vi "DynamicHoppingScan.vi"() -> ()   [LabVIEW 2014]
uses:
  <vilib>/userdefined/High Color/nirio_resource_hc.ctl
  <vilib>/Instr/_visa.llb/VISA Configure Serial Port (Instr).vi
  <vilib>/FPGAPlugInAG/PCIe-7851R/niLvFpga_Open_PCIe-7851R.vi
  <vilib>/rvi/interface/common/dynamic/niFpgaDynamicAddResources.vi
  <vilib>/Utility/error.llb/Error Cluster From Error Code.vi
  <vilib>/rvi/errors/niLvFpgaAdjustHostInterfaceError.vi
  <vilib>/FPGAPlugInAG/Dynamic/niLvFpga_Close_Dynamic.vi
  <vilib>/rvi/interface/nirviOpenFPGA/nirviOpenFPGA.xnode
  FPGATest_FPGATarget_PIZApproaching_ngy2QjQf4ns.lvbitx
  <vilib>/rvi/interface/nirviReadWriteControl/nirviReadWriteControl.xnode
  <vilib>/rvi/interface/nirviCloseFPGA/nirviCloseFPGA.xnode
  FPGATest_FPGATarget_PIZWithdraw_LXoQbY-wYvI.lvbitx
  <vilib>/rvi/interface/Simulation/niFpgaSimulationCallBeginRW.vi
  NiFpgaLv.dll
  NextXYPos.dll
panel:
  out "RoughXYZErr?":string
  out "XY Graph":cluster{dbl[], dbl[]}(graph)
  in  "stepMultiplier / 0.305nm":i16
  out "preCurrIndexDia":i16(graph)
  out "PIZPosDia":i16(graph)
  out "PIZPos":i16
  out "preCurrIndex":i16
  out "refCurrIndex":i16
  in  "stop":bool
  in  "ThresholdIndex":i32
  in  "PIZ":T1
  in  "PIZRisingLimitLen / um":dbl
  out "YPos?":dbl
  out "XPos?":dbl
  in  "YIStep / um":dbl format="%#_13g"
  in  "XIStep / um":dbl format="%#_13g"
  in  "YDirTotalLength / um":dbl format="%#_13g"
  in  "XDirTotalLength / um":dbl format="%#_13g"
  in  "Y Init / um":dbl format="%#_13g"
  in  "X Init / um":dbl format="%#_13g"
  in  "AllLoopSleep ms":i32
  in  "RoughXYZ":refnum<visa-resource-name>
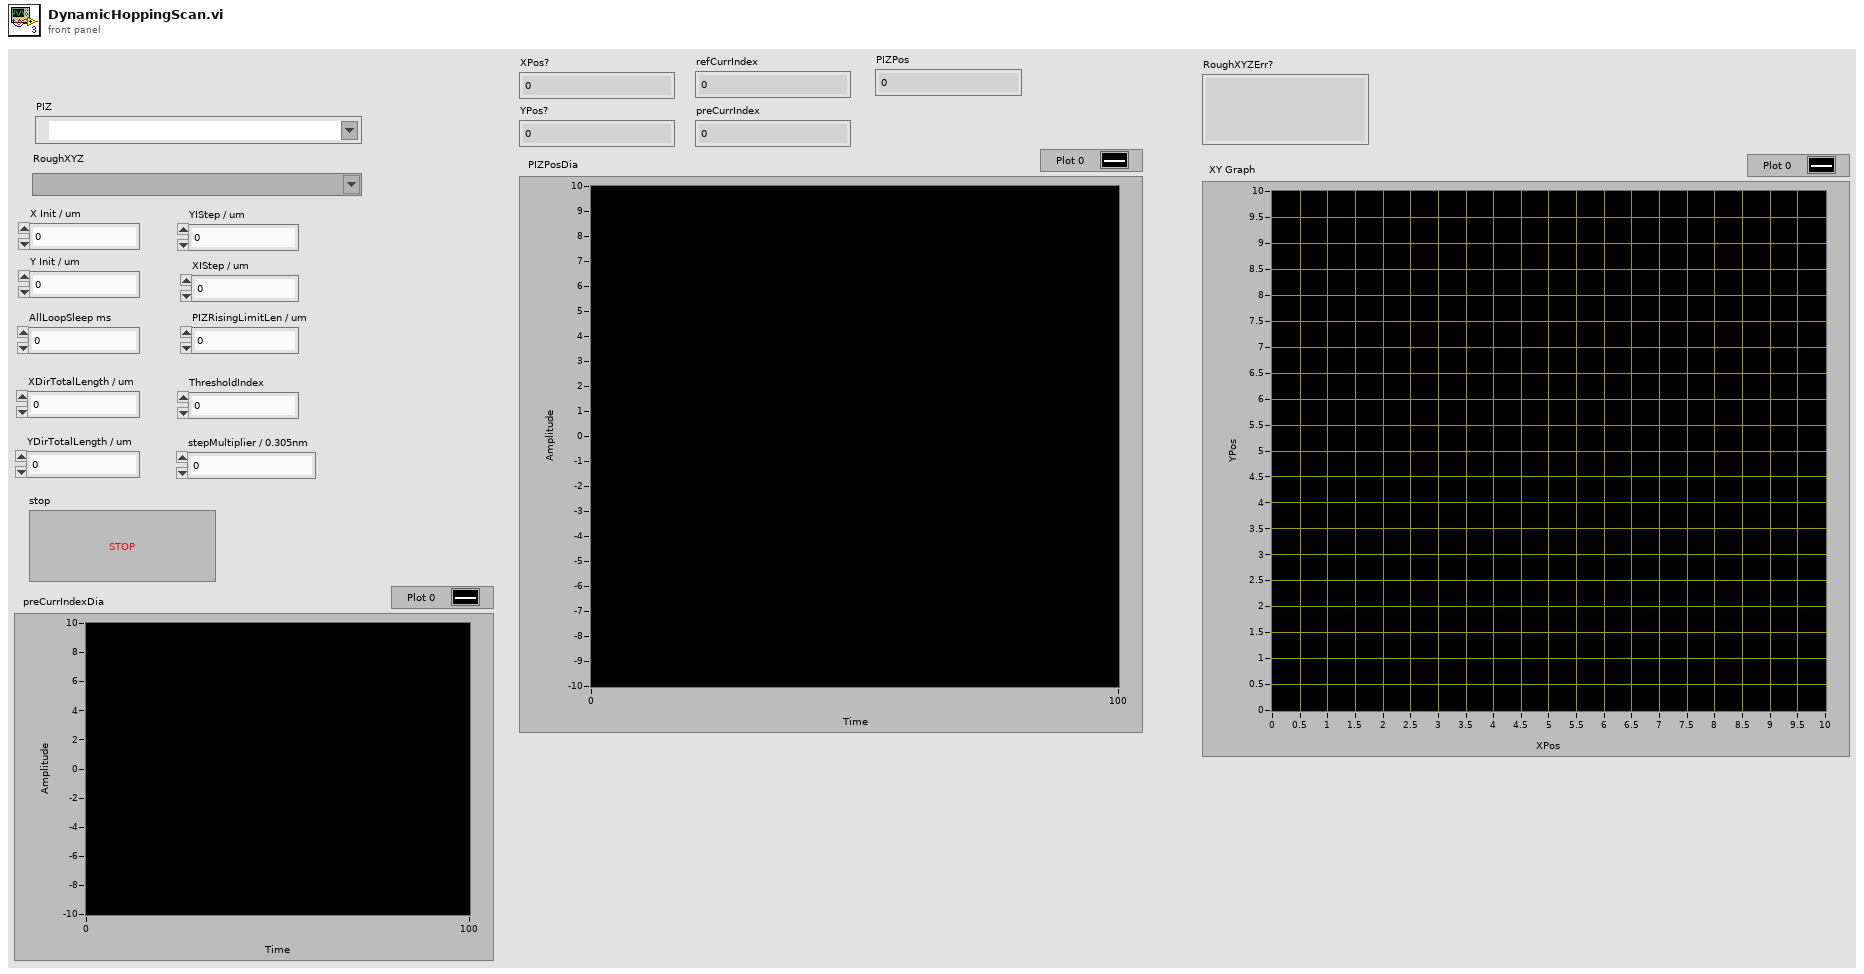
[diagram p1: front panel]
types:
  T1 = typedef "nirio_resource_hc.ctl" = tag
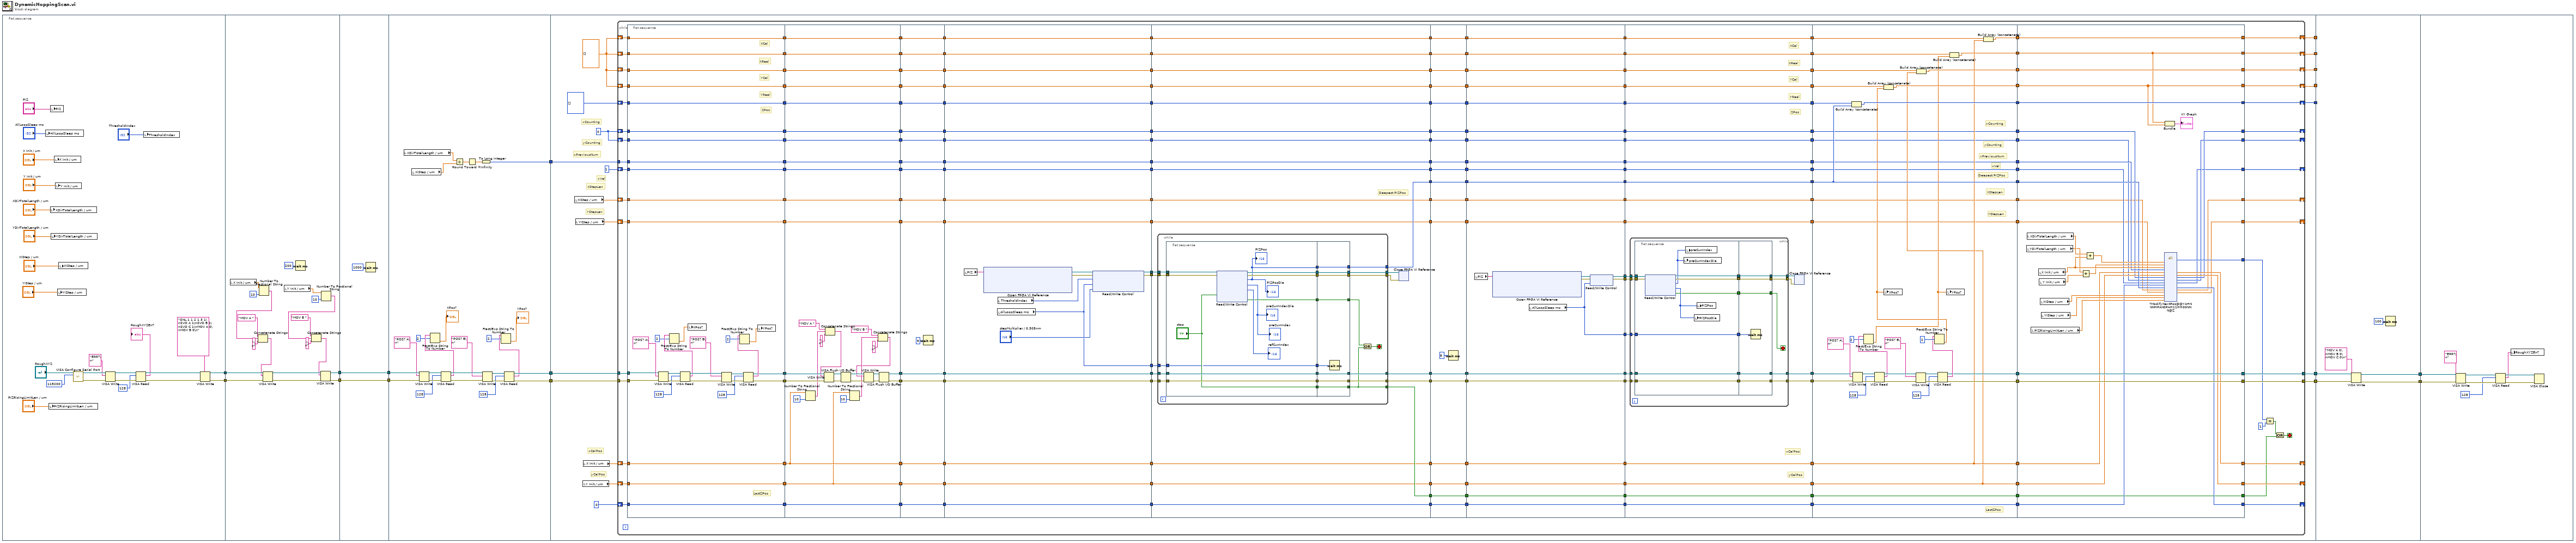
[diagram p0: block diagram]
diagram:
  n1 = flat-sequence {
    tunnel: [w35] -> w18
    tunnel: [w34] -> w17
    tunnel: w18 -> [w60]
    tunnel: w17 -> [w59]
    tunnel: [w44] -> w16
    tunnel: [w43] -> w15
    tunnel: w16 -> [w63]
    tunnel: w15 -> [w62]
    tunnel: [w63] -> w14
    tunnel: [w62] -> w13
    tunnel: w14 -> [w89]
    tunnel: w13 -> [w88]
    tunnel: [w77] -> w12
    tunnel: [w76] -> w11
    tunnel: [w65] -> w10
    tunnel: w12 -> [w108]
    tunnel: w11 -> [w107]
    tunnel: w10 -> [w106]
    tunnel: [w105] -> w9
    tunnel: [w104] -> w8
    tunnel: [w103] -> w7
    tunnel: [w102] -> w6
    tunnel: [w100] -> w5
    tunnel: [w91] -> w4
    tunnel: [w90] -> w3
    tunnel: w9 -> [_]
    tunnel: w8 -> [_]
    tunnel: w7 -> [_]
    tunnel: w6 -> [_]
    tunnel: w5 -> [_]
    tunnel: w4 -> [w663]
    tunnel: w3 -> [w662]
    tunnel: [w660] -> w2
    tunnel: [w659] -> w1
    tunnel: w2 -> [w672]
    tunnel: w1 -> [w671]
    frame #0 {
      n2 = local write "AllLoopSleep ms"("AllLoopSleep ms") -> ()
      n3 = local write "PIZRisingLimitLen / um"("PIZRisingLimitLen / um") -> ()
      n4 = local write "XDirTotalLength / um"("XDirTotalLength / um") -> ()
      n5 = local write "PIZ"("PIZ") -> ()
      n6 = local write "YDirTotalLength / um"("YDirTotalLength / um") -> ()
      n7 = local write "X Init / um"("X Init / um") -> ()
      n8 = local write "Y Init / um"("Y Init / um") -> ()
      n9 = local write "YIStep / um"("YIStep / um") -> ()
      n10 = local write "XIStep / um"("XIStep / um") -> ()
      n11 = call-poly "VISA Configure Serial Port"("VISA resource name"="RoughXYZ", "baud rate (9600)"=u32 115200) -> ("VISA resource name out"=w40:refnum<visa-resource-name>, "error out"=w39:errorcluster)  [unwired: 12 in]
      n12 = VISA Write(VISA resource name=w40, write buffer="ERR?\n", error in (no error)=w39) -> (VISA resource name out=w24:refnum<visa-resource-name>, error out=w23:errorcluster)  [unwired: 1 out]
      n13 = VISA Read(VISA resource name=w24, byte count=u32 128, error in (no error)=w23) -> (VISA resource name out=w22:refnum<visa-resource-name>, read buffer=→"RoughXYZErr?":string, error out=w21:errorcluster)  [unwired: 1 out]
      n14 = local write "ThresholdIndex"("ThresholdIndex") -> ()
      n15 = VISA Write(VISA resource name=w22, write buffer="ONL 1 1 2 1 3 1\nSVO A 1\nSVO B 1\nSVO C 1\nMOV A 0\nMOV B 0\n", error in (no error)=w21) -> (VISA resource name out=w35:refnum<visa-resource-name>, error out=w34:errorcluster)  [unwired: 1 out]
    }
    frame #1 {
      n16 = local read "X Init / um"() -> (w56:dbl)
      n17 = Number To Fractional String(number=w56, precision (6)=i16 10) -> (F-format string=w54:string)  [unwired: 2 in]
      n18 = Concatenate Strings("MOV A " ("string"), w54, "\n" ("string")) -> (w58:string)
      n19 = VISA Write(VISA resource name=w60, write buffer=w58, error in (no error)=w59) -> (VISA resource name out=w52:refnum<visa-resource-name>, error out=w51:errorcluster)  [unwired: 1 out]
      n20 = local read "Y Init / um"() -> (w50:dbl)
      n21 = Wait (ms)(milliseconds to wait=u32 200) -> ()  [unwired: 1 out]
      n22 = Number To Fractional String(number=w50, precision (6)=i16 10) -> (F-format string=w45:string)  [unwired: 2 in]
      n23 = Concatenate Strings("MOV B " ("string"), w45, "\n" ("string")) -> (w46:string)
      n24 = VISA Write(VISA resource name=w52, write buffer=w46, error in (no error)=w51) -> (VISA resource name out=w44:refnum<visa-resource-name>, error out=w43:errorcluster)  [unwired: 1 out]
    }
    frame #2 {
      n25 = Wait (ms)(milliseconds to wait=u32 1000) -> ()  [unwired: 1 out]
    }
    frame #3 {
      n26 = local read "XDirTotalLength / um"() -> (w69:dbl)
      n27 = local read "XIStep / um"() -> (w68:dbl)
      n28 = VISA Write(VISA resource name=w89, write buffer="POS? A\n", error in (no error)=w88) -> (VISA resource name out=w86:refnum<visa-resource-name>, error out=w85:errorcluster)  [unwired: 1 out]
      n29 = VISA Read(VISA resource name=w86, byte count=u32 128, error in (no error)=w85) -> (VISA resource name out=w80:refnum<visa-resource-name>, read buffer=w75:string, error out=w79:errorcluster)  [unwired: 1 out]
      n30 = Fract/Exp String To Number(string=w75, offset=2) -> (number=→"XPos?":dbl)  [unwired: 2 in, 1 out]
      n31 = Divide(x=w69, y=w68) -> (x/y=w67:dbl)
      n32 = Round Toward +Infinity(x=w67) -> (ceil(x): smallest int >= x=w66:dbl)
      n33 = To Long Integer(number=w66) -> (32bit integer=w65:i32)
      n34 = VISA Write(VISA resource name=w80, write buffer="POS? B\n", error in (no error)=w79) -> (VISA resource name out=w83:refnum<visa-resource-name>, error out=w82:errorcluster)  [unwired: 1 out]
      n35 = VISA Read(VISA resource name=w83, byte count=u32 128, error in (no error)=w82) -> (VISA resource name out=w77:refnum<visa-resource-name>, read buffer=w70:string, error out=w76:errorcluster)  [unwired: 1 out]
      n36 = Fract/Exp String To Number(string=w70, offset=2) -> (number=→"YPos?":dbl)  [unwired: 2 in, 1 out]
    }
    frame #4 {
      w101 = dbl[] []
      w98 = 0
      # "yCalPos"
      # "xCalPos"
      # "YStepLen"
      # "XStepLen"
      # "xVel"
      # "xPreviousNum"
      # "yCounting"
      # "xCounting"
      n37 = local read "XIStep / um"() -> (w96:dbl)
      n38 = local read "YIStep / um"() -> (w95:dbl)
      n39 = local read "Y Init / um"() -> (w93:dbl)
      n40 = local read "X Init / um"() -> (w94:dbl)
      n41 = while {
        tunnel: w108 -> [w304]
        tunnel: w107 -> [w303]
        tunnel: w106 -> [w302]
        shift-right: [w141] -> w105
        shift-left: w101 -> [w138]
        shift-right: [w137] -> w102
        shift-left: w101 -> [w243]
        shift-right: [w140] -> w104
        shift-left: w101 -> [w136]
        shift-right: [w135] -> w100
        shift-left: w101 -> [w240]
        shift-right: [w139] -> w103
        shift-left: i32[] [] -> [w134]
        tunnel: [w128] -> w91
        tunnel: [w127] -> w90
        shift-right: [w133] -> _
        shift-left: w98 -> [w123]
        shift-right: [w132] -> _
        shift-left: w98 -> [w122]
        shift-right: [w131] -> _
        shift-left: 1 ("xVel") -> [w121]
        shift-right: [w130] -> _
        shift-left: w96 -> [w120]
        shift-right: [w129] -> _
        shift-left: w95 -> [w119]
        shift-right: [w126] -> _
        shift-left: w94 -> [w118]
        shift-right: [w125] -> _
        shift-left: w93 -> [w117]
        shift-right: [w124] -> _
        shift-left: 0 -> [w116]
        stop <- w115 stop-if-true
        n42 = flat-sequence {
          tunnel: w304 -> [w324]
          tunnel: w303 -> [w323]
          tunnel: w123 -> [w310]
          tunnel: w122 -> [w311]
          tunnel: w302 -> [w312]
          tunnel: w121 -> [w313]
          tunnel: w120 -> [w314]
          tunnel: w119 -> [w315]
          tunnel: [w322] -> w301
          tunnel: [w321] -> w300
          tunnel: w116 -> [w318]
          tunnel: [w318] -> w299
          tunnel: w118 -> [w317]
          tunnel: w117 -> [w316]
          tunnel: [w317] -> w298
          tunnel: [w316] -> w297
          tunnel: [w315] -> w294
          tunnel: [w314] -> w293
          tunnel: [w313] -> w292
          tunnel: [w312] -> w291
          tunnel: [w311] -> w290
          tunnel: [w310] -> w289
          tunnel: [w309] -> w245
          tunnel: w138 -> [w309]
          tunnel: [w308] -> w244
          tunnel: w243 -> [w308]
          tunnel: [w307] -> w242
          tunnel: w136 -> [w307]
          tunnel: [w306] -> w241
          tunnel: w240 -> [w306]
          tunnel: w134 -> [w305]
          tunnel: [w305] -> w235
          tunnel: w301 -> [w372]
          tunnel: w300 -> [w371]
          tunnel: w299 -> [w339]
          tunnel: w298 -> [w341]
          tunnel: w297 -> [w340]
          tunnel: [w354] -> w296
          tunnel: [w353] -> w295
          tunnel: w294 -> [w352]
          tunnel: w293 -> [w351]
          tunnel: w292 -> [w350]
          tunnel: w291 -> [w349]
          tunnel: w290 -> [w348]
          tunnel: w289 -> [w347]
          tunnel: [w352] -> w288
          tunnel: [w351] -> w287
          tunnel: [w350] -> w286
          tunnel: [w349] -> w285
          tunnel: [w348] -> w284
          tunnel: [w347] -> w283
          tunnel: w245 -> [w346]
          tunnel: w244 -> [w345]
          tunnel: w242 -> [w344]
          tunnel: w241 -> [w343]
          tunnel: [w346] -> w239
          tunnel: [w345] -> w238
          tunnel: [w344] -> w237
          tunnel: [w343] -> w236
          tunnel: w235 -> [w342]
          tunnel: [w342] -> w234
          tunnel: [w341] -> w203
          tunnel: [w340] -> w202
          tunnel: [w339] -> w201
          tunnel: w296 -> [w388]
          tunnel: w295 -> [w387]
          tunnel: [w388] -> w282
          tunnel: [w387] -> w280
          tunnel: w288 -> [w386]
          tunnel: w287 -> [w385]
          tunnel: w286 -> [w384]
          tunnel: w285 -> [w383]
          tunnel: w284 -> [w382]
          tunnel: w283 -> [w381]
          tunnel: [w386] -> w274
          tunnel: [w385] -> w272
          tunnel: [w384] -> w269
          tunnel: [w383] -> w266
          tunnel: [w382] -> w263
          tunnel: [w381] -> w260
          tunnel: w239 -> [w380]
          tunnel: w238 -> [w379]
          tunnel: w237 -> [w378]
          tunnel: w236 -> [w377]
          tunnel: w234 -> [w376]
          tunnel: [w380] -> w233
          tunnel: [w379] -> w232
          tunnel: [w378] -> w231
          tunnel: [w377] -> w230
          tunnel: [w376] -> w229
          tunnel: w203 -> [w373]
          tunnel: w202 -> [w374]
          tunnel: w201 -> [w375]
          tunnel: [w375] -> w200
          tunnel: [w374] -> w199
          tunnel: [w373] -> w198
          tunnel: w282 -> [w413]
          tunnel: [w413] -> w281
          tunnel: w280 -> [w412]
          tunnel: [w412] -> w279
          tunnel: [w407] -> w278
          tunnel: [w406] -> w277
          tunnel: [w405] -> w275
          tunnel: w274 -> [w405]
          tunnel: [w404] -> w273
          tunnel: w272 -> [w404]
          tunnel: [w403] -> w270
          tunnel: w269 -> [w403]
          tunnel: [w402] -> w267
          tunnel: w266 -> [w402]
          tunnel: [w401] -> w264
          tunnel: w263 -> [w401]
          tunnel: [w400] -> w261
          tunnel: w260 -> [w400]
          tunnel: w233 -> [w394]
          tunnel: w232 -> [w395]
          tunnel: w231 -> [w396]
          tunnel: w230 -> [w397]
          tunnel: w229 -> [w398]
          tunnel: [w398] -> w228
          tunnel: [w397] -> w227
          tunnel: [w396] -> w226
          tunnel: [w395] -> w225
          tunnel: [w394] -> w224
          tunnel: w200 -> [w391]
          tunnel: w199 -> [w392]
          tunnel: w198 -> [w393]
          tunnel: [w393] -> w197
          tunnel: [w392] -> w196
          tunnel: [w391] -> w195
          tunnel: [w390] -> w110
          tunnel: w281 -> [w438]
          tunnel: w279 -> [w437]
          tunnel: w278 -> [w436]
          tunnel: w277 -> [w435]
          tunnel: [w432] -> w276
          tunnel: w275 -> [w426]
          tunnel: w273 -> [w427]
          tunnel: [w431] -> w271
          tunnel: w270 -> [w431]
          tunnel: [w430] -> w268
          tunnel: w267 -> [w430]
          tunnel: [w429] -> w265
          tunnel: w264 -> [w429]
          tunnel: [w428] -> w262
          tunnel: w261 -> [w428]
          tunnel: [w427] -> w259
          tunnel: [w426] -> w258
          tunnel: [w425] -> w257
          tunnel: [w424] -> w251
          tunnel: [w423] -> w248
          tunnel: w228 -> [w422]
          tunnel: w227 -> [w421]
          tunnel: w226 -> [w420]
          tunnel: w225 -> [w419]
          tunnel: w224 -> [w418]
          tunnel: [w422] -> w222
          tunnel: [w421] -> w220
          tunnel: [w420] -> w218
          tunnel: [w419] -> w216
          tunnel: [w418] -> w214
          tunnel: w197 -> [w417]
          tunnel: w196 -> [w416]
          tunnel: w195 -> [w415]
          tunnel: [w417] -> w193
          tunnel: [w416] -> w191
          tunnel: [w415] -> w189
          tunnel: w110 -> [w414]
          tunnel: w276 -> [w484]
          tunnel: w271 -> [w483]
          tunnel: w268 -> [w482]
          tunnel: w265 -> [w481]
          tunnel: w262 -> [w480]
          tunnel: w259 -> [w485]
          tunnel: w258 -> [w486]
          tunnel: w257 -> [w497]
          tunnel: [w497] -> w256
          tunnel: [w496] -> w252
          tunnel: w251 -> [w496]
          tunnel: [w495] -> w249
          tunnel: w248 -> [w495]
          tunnel: [w494] -> w223
          tunnel: w222 -> [w494]
          tunnel: [w493] -> w221
          tunnel: w220 -> [w493]
          tunnel: [w492] -> w219
          tunnel: w218 -> [w492]
          tunnel: [w491] -> w217
          tunnel: w216 -> [w491]
          tunnel: [w490] -> w215
          tunnel: w214 -> [w490]
          tunnel: [w489] -> w194
          tunnel: w193 -> [w489]
          tunnel: [w488] -> w192
          tunnel: w191 -> [w488]
          tunnel: [w487] -> w190
          tunnel: w189 -> [w487]
          tunnel: [w486] -> w175
          tunnel: [w485] -> w172
          tunnel: [w484] -> w169
          tunnel: [w483] -> w166
          tunnel: [w482] -> w163
          tunnel: [w481] -> w160
          tunnel: [w480] -> w157
          tunnel: w256 -> [w500]
          tunnel: [w519] -> w255
          tunnel: [w518] -> w254
          tunnel: [w517] -> w253
          tunnel: w252 -> [w517]
          tunnel: [w516] -> w250
          tunnel: w249 -> [w516]
          tunnel: w223 -> [w515]
          tunnel: w221 -> [w514]
          tunnel: w219 -> [w513]
          tunnel: w217 -> [w512]
          tunnel: w215 -> [w511]
          tunnel: [w515] -> w213
          tunnel: [w514] -> w212
          tunnel: [w513] -> w211
          tunnel: [w512] -> w210
          tunnel: [w511] -> w209
          tunnel: w194 -> [w510]
          tunnel: w192 -> [w509]
          tunnel: w190 -> [w508]
          tunnel: [w510] -> w187
          tunnel: [w509] -> w186
          tunnel: [w508] -> w183
          tunnel: [w507] -> w176
          tunnel: w175 -> [w507]
          tunnel: [w506] -> w173
          tunnel: w172 -> [w506]
          tunnel: [w505] -> w170
          tunnel: w169 -> [w505]
          tunnel: [w504] -> w167
          tunnel: w166 -> [w504]
          tunnel: [w503] -> w164
          tunnel: w163 -> [w503]
          tunnel: [w502] -> w161
          tunnel: w160 -> [w502]
          tunnel: [w501] -> w158
          tunnel: w157 -> [w501]
          tunnel: [w500] -> w149
          tunnel: [w499] -> w109
          tunnel: w255 -> [w547]
          tunnel: w254 -> [w546]
          tunnel: w253 -> [w543]
          tunnel: w250 -> [w542]
          tunnel: [w541] -> w247
          tunnel: [w540] -> w246
          tunnel: w213 -> [w539]
          tunnel: w212 -> [w538]
          tunnel: w211 -> [w537]
          tunnel: w210 -> [w536]
          tunnel: w209 -> [w535]
          tunnel: [w539] -> w208
          tunnel: [w538] -> w207
          tunnel: [w537] -> w206
          tunnel: [w536] -> w205
          tunnel: [w535] -> w204
          tunnel: [w534] -> w188
          tunnel: w187 -> [w534]
          tunnel: w186 -> [w533]
          tunnel: [w533] -> w185
          tunnel: [w532] -> w184
          tunnel: w183 -> [w532]
          tunnel: [w531] -> w177
          tunnel: w176 -> [w531]
          tunnel: [w530] -> w174
          tunnel: w173 -> [w530]
          tunnel: [w529] -> w171
          tunnel: w170 -> [w529]
          tunnel: [w528] -> w168
          tunnel: w167 -> [w528]
          tunnel: [w527] -> w165
          tunnel: w164 -> [w527]
          tunnel: [w526] -> w162
          tunnel: w161 -> [w526]
          tunnel: [w525] -> w159
          tunnel: w158 -> [w525]
          tunnel: [w524] -> w150
          tunnel: w149 -> [w524]
          tunnel: w109 -> [w523]
          tunnel: w247 -> [w606]
          tunnel: w246 -> [w605]
          tunnel: w208 -> [w601]
          tunnel: w207 -> [w600]
          tunnel: w206 -> [w599]
          tunnel: w205 -> [w598]
          tunnel: w204 -> [w597]
          tunnel: w188 -> [w590]
          tunnel: w185 -> [w589]
          tunnel: w184 -> [w604]
          tunnel: [w590] -> w182
          tunnel: [w589] -> w181
          tunnel: [w604] -> w180
          tunnel: [w603] -> w179
          tunnel: [w602] -> w178
          tunnel: w177 -> [w582]
          tunnel: w174 -> [w583]
          tunnel: w171 -> [w596]
          tunnel: w168 -> [w584]
          tunnel: w165 -> [w585]
          tunnel: w162 -> [w586]
          tunnel: w159 -> [w587]
          tunnel: [w596] -> w156
          tunnel: [w595] -> w155
          tunnel: [w594] -> w154
          tunnel: [w593] -> w153
          tunnel: [w592] -> w152
          tunnel: [w591] -> w151
          tunnel: w150 -> [w588]
          tunnel: [w588] -> w148
          tunnel: [w587] -> w147
          tunnel: [w586] -> w146
          tunnel: [w585] -> w145
          tunnel: [w584] -> w144
          tunnel: [w583] -> w143
          tunnel: [w582] -> w142
          tunnel: [w657] -> w141
          tunnel: [w622] -> w137
          tunnel: [w656] -> w140
          tunnel: [w621] -> w135
          tunnel: [w655] -> w139
          tunnel: w142 -> [w626]
          tunnel: w143 -> [w628]
          tunnel: w144 -> [w632]
          tunnel: w145 -> [w648]
          tunnel: w146 -> [w634]
          tunnel: w147 -> [w636]
          tunnel: w148 -> [w624]
          tunnel: w151 -> [w657]
          tunnel: w152 -> [w622]
          tunnel: w153 -> [w656]
          tunnel: w154 -> [w621]
          tunnel: w155 -> [w655]
          tunnel: w156 -> [w647]
          tunnel: w178 -> [w642]
          tunnel: w179 -> [w643]
          tunnel: w180 -> [w630]
          tunnel: w181 -> [w638]
          tunnel: w182 -> [w640]
          tunnel: [w643] -> w128
          tunnel: [w642] -> w127
          tunnel: [w641] -> w111
          tunnel: [w639] -> w126
          tunnel: [w637] -> w125
          tunnel: [w633] -> w132
          tunnel: [w635] -> w133
          tunnel: [w631] -> w131
          tunnel: [w629] -> w124
          tunnel: [w627] -> w130
          tunnel: [w625] -> w129
          tunnel: [w624] -> w114
          frame #0 {
            # "ZPos"
            # "YReal"
            # "YCal"
            # "XReal"
            # "XCal"
            # "LastZPos"
            n43 = VISA Write(VISA resource name=w324, write buffer="POS? A\n", error in (no error)=w323) -> (VISA resource name out=w337:refnum<visa-resource-name>, error out=w336:errorcluster)  [unwired: 1 out]
            n44 = VISA Read(VISA resource name=w337, byte count=u32 128, error in (no error)=w336) -> (VISA resource name out=w331:refnum<visa-resource-name>, read buffer=w328:string, error out=w330:errorcluster)  [unwired: 1 out]
            n45 = Fract/Exp String To Number(string=w328, offset=2) -> (number=w319:dbl)  [unwired: 2 in, 1 out]
            n46 = local write "XPos?"(w319) -> ()
            n47 = VISA Write(VISA resource name=w331, write buffer="POS? B\n", error in (no error)=w330) -> (VISA resource name out=w334:refnum<visa-resource-name>, error out=w333:errorcluster)  [unwired: 1 out]
            n48 = VISA Read(VISA resource name=w334, byte count=u32 128, error in (no error)=w333) -> (VISA resource name out=w322:refnum<visa-resource-name>, read buffer=w325:string, error out=w321:errorcluster)  [unwired: 1 out]
            n49 = Fract/Exp String To Number(string=w325, offset=2) -> (number=w320:dbl)  [unwired: 2 in, 1 out]
            n50 = local write "YPos?"(w320) -> ()
          }
          frame #1 {
            n51 = Number To Fractional String(number=w341, precision (6)=i16 10) -> (F-format string=w363:string)  [unwired: 2 in]
            n52 = Concatenate Strings("MOV A " ("string"), w363, "\n" ("string")) -> (w360:string)
            n53 = VISA Write(VISA resource name=w372, write buffer=w360, error in (no error)=w371) -> (VISA resource name out=w369:refnum<visa-resource-name>, error out=w370:errorcluster)  [unwired: 1 out]
            n54 = VISA Flush I/O Buffer(VISA resource name=w369, error in (no error)=w370) -> (VISA resource name out=w368:refnum<visa-resource-name>, error out=w367:errorcluster)  [unwired: 1 in]
            n55 = Number To Fractional String(number=w340, precision (6)=i16 10) -> (F-format string=w356:string)  [unwired: 2 in]
            n56 = Concatenate Strings("MOV B " ("string"), w356, "\n" ("string")) -> (w355:string)
            n57 = VISA Write(VISA resource name=w368, write buffer=w355, error in (no error)=w367) -> (VISA resource name out=w366:refnum<visa-resource-name>, error out=w365:errorcluster)  [unwired: 1 out]
            n58 = VISA Flush I/O Buffer(VISA resource name=w366, error in (no error)=w365) -> (VISA resource name out=w354:refnum<visa-resource-name>, error out=w353:errorcluster)  [unwired: 1 in]
          }
          frame #2 {
            n59 = Wait (ms)(milliseconds to wait=u32 5) -> ()  [unwired: 1 out]
          }
          frame #3 {
            n60 = local read "PIZ"() -> (w408:T1)
            n61 = xnode "Open FPGA VI Reference"("resource name"=w408) -> ("FPGA VI Reference Out"=w409:refnum<k20>, "error out"=w410:errorcluster)  [unwired: 1 in]
            n62 = local read "AllLoopSleep ms"() -> (w390:i32)
            n63 = local read "ThresholdIndex"() -> (w411:i32)
            n64 = xnode "Read/Write Control"("FPGA VI Reference In"=w409, "error in"=w410, "thresholdIndex"=w411, "Sleep ms"=w390, "stepMultiplier / 0.305nm"="stepMultiplier / 0.305nm") -> ("FPGA VI Reference Out"=w407:refnum<k20>, "error out"=w406:errorcluster)
          }
          frame #4 {
            # "Deepest PIZPos"
            n65 = while {
              tunnel: w438 -> [w459]
              tunnel: w437 -> [w458]
              tunnel: w436 -> [w454]
              tunnel: w435 -> [w453]
              tunnel: [w450] -> w433
              tunnel: [w449] -> w434
              tunnel: [w447] -> w424
              tunnel: [w446] -> w423
              tunnel: [w442] -> w432
              tunnel: [w441] -> w425
              tunnel: w414 -> [w440]
              stop <- w448 stop-if-true
              n66 = flat-sequence {
                tunnel: w459 -> [w471]
                tunnel: w458 -> [w470]
                tunnel: ["stop"] -> w457
                tunnel: [w471] -> w456
                tunnel: [w470] -> w455
                tunnel: w454 -> [w469]
                tunnel: w453 -> [w468]
                tunnel: [w466] -> w452
                tunnel: [w465] -> w451
                tunnel: [w463] -> w445
                tunnel: [w461] -> w443
                tunnel: w440 -> [w460]
                tunnel: [w460] -> w439
                tunnel: w457 -> [w479]
                tunnel: [w479] -> w441
                tunnel: w456 -> [w476]
                tunnel: w455 -> [w475]
                tunnel: w452 -> [w478]
                tunnel: w451 -> [w477]
                tunnel: [w478] -> w449
                tunnel: [w477] -> w450
                tunnel: [w476] -> w447
                tunnel: [w475] -> w446
                tunnel: w445 -> [w474]
                tunnel: [w474] -> w444
                tunnel: w443 -> [w473]
                tunnel: [w473] -> w442
                tunnel: w439 -> [w472]
                frame #0 {
                  n67 = xnode "Read/Write Control"("FPGA VI Reference In"=w469, "error in"=w468, "stop"="stop") -> ("FPGA VI Reference Out"=w466:refnum<k20>, "error out"=w465:errorcluster, "PIZPos"=w461:i16, "preCurrIndex"=→"preCurrIndex" →"preCurrIndexDia":i16, "refCurrIndex"=→"refCurrIndex":i16, "Approached?"=w463:bool)
                  "PIZPos" <- w461
                  "PIZPosDia" <- w461
                }
                frame #1 {
                  n68 = Wait (ms)(milliseconds to wait=w472) -> ()  [unwired: 1 out]
                }
              }
              n69 = Or(x=w444, y=w441) -> (x .or. y?=w448:bool)
            }
            n70 = xnode "Close FPGA VI Reference"("FPGA VI Reference In"=w434, "error in"=w433) -> ()  [unwired: 1 out]
          }
          frame #5 {
            n71 = Wait (ms)(milliseconds to wait=u32 5) -> ()  [unwired: 1 out]
          }
          frame #6 {
            n72 = local read "PIZ"() -> (w522:T1)
            n73 = xnode "Open FPGA VI Reference"("resource name"=w522) -> ("FPGA VI Reference Out"=w521:refnum<k20>, "error out"=w520:errorcluster)  [unwired: 1 in]
            n74 = local read "AllLoopSleep ms"() -> (w499:i32)
            n75 = xnode "Read/Write Control"("FPGA VI Reference In"=w521, "error in"=w520, "Sleep ms"=w499) -> ("FPGA VI Reference Out"=w519:refnum<k20>, "error out"=w518:errorcluster)
          }
          frame #7 {
            # "yCalPos"
            # "xCalPos"
            # "ZPos"
            # "YReal"
            # "YCal"
            # "XReal"
            # "XCal"
            n76 = while {
              tunnel: w547 -> [w563]
              tunnel: w546 -> [w562]
              tunnel: [w557] -> w545
              tunnel: [w556] -> w544
              tunnel: w543 -> [w554]
              tunnel: w542 -> [w552]
              tunnel: [w551] -> w541
              tunnel: [w550] -> w540
              tunnel: w523 -> [w548]
              stop <- w558 stop-if-true
              n77 = flat-sequence {
                tunnel: w563 -> [w573]
                tunnel: w562 -> [w572]
                tunnel: [w571] -> w561
                tunnel: [w570] -> w560
                tunnel: [w567] -> w559
                tunnel: [w566] -> w555
                tunnel: w554 -> [w566]
                tunnel: [w565] -> w553
                tunnel: w552 -> [w565]
                tunnel: [w564] -> w549
                tunnel: w548 -> [w564]
                tunnel: w561 -> [w578]
                tunnel: w560 -> [w577]
                tunnel: w559 -> [w579]
                tunnel: [w579] -> w558
                tunnel: [w578] -> w557
                tunnel: [w577] -> w556
                tunnel: w555 -> [w576]
                tunnel: w553 -> [w575]
                tunnel: [w576] -> w551
                tunnel: [w575] -> w550
                tunnel: w549 -> [w574]
                frame #0 {
                  n78 = xnode "Read/Write Control"("FPGA VI Reference In"=w573, "error in"=w572) -> ("FPGA VI Reference Out"=w571:refnum<k20>, "error out"=w570:errorcluster, "preCurrIndex"=w569:i16, "PIZPos?"=w568:i16, "Withdrawn?"=w567:bool)
                  n79 = local write "preCurrIndexDia"(w569) -> ()
                  n80 = local write "preCurrIndex"(w569) -> ()
                  n81 = local write "PIZPosDia"(w568) -> ()
                  n82 = local write "PIZPos"(w568) -> ()
                }
                frame #1 {
                  n83 = Wait (ms)(milliseconds to wait=w574) -> ()  [unwired: 1 out]
                }
              }
            }
            n84 = xnode "Close FPGA VI Reference"("FPGA VI Reference In"=w545, "error in"=w544) -> ()  [unwired: 1 out]
          }
          frame #8 {
            # "LastZPos"
            # "Deepest PIZPos"
            # "YStepLen"
            # "XStepLen"
            # "xVel"
            # "xPreviousNum"
            # "yCounting"
            # "xCounting"
            n85 = Build Array (concatenate)(w601, w596) -> (w595:i32[])
            n86 = VISA Write(VISA resource name=w606, write buffer="POS? A\n", error in (no error)=w605) -> (VISA resource name out=w619:refnum<visa-resource-name>, error out=w618:errorcluster)  [unwired: 1 out]
            n87 = VISA Read(VISA resource name=w619, byte count=u32 128, error in (no error)=w618) -> (VISA resource name out=w613:refnum<visa-resource-name>, read buffer=w610:string, error out=w612:errorcluster)  [unwired: 1 out]
            n88 = Fract/Exp String To Number(string=w610, offset=2) -> (number=w580:dbl)  [unwired: 2 in, 1 out]
            n89 = VISA Write(VISA resource name=w613, write buffer="POS? B\n", error in (no error)=w612) -> (VISA resource name out=w616:refnum<visa-resource-name>, error out=w615:errorcluster)  [unwired: 1 out]
            n90 = Build Array (concatenate)(w599, w589) -> (w593:dbl[])
            n91 = VISA Read(VISA resource name=w616, byte count=u32 128, error in (no error)=w615) -> (VISA resource name out=w603:refnum<visa-resource-name>, read buffer=w607:string, error out=w602:errorcluster)  [unwired: 1 out]
            n92 = Fract/Exp String To Number(string=w607, offset=2) -> (number=w581:dbl)  [unwired: 2 in, 1 out]
            n93 = local write "XPos?"(w581) -> ()
            n94 = Build Array (concatenate)(w600, w581) -> (w594:dbl[])
            n95 = local write "YPos?"(w580) -> ()
            n96 = Build Array (concatenate)(w598, w580) -> (w592:dbl[])
            n97 = Build Array (concatenate)(w597, w590) -> (w591:dbl[])
          }
          frame #9 {
            n98 = local read "YDirTotalLength / um"() -> (w651:dbl)
            n99 = local read "XDirTotalLength / um"() -> (w654:dbl)
            n100 = local read "PIZRisingLimitLen / um"() -> (w644:dbl)
            n101 = local read "X Init / um"() -> (w653:dbl)
            n102 = local read "Y Init / um"() -> (w650:dbl)
            n103 = local read "XIStep / um"() -> (w646:dbl)
            n104 = local read "YIStep / um"() -> (w645:dbl)
            n105 = Add(x=w651, y=w650) -> (x+y=w649:dbl)
            n106 = Add(x=w654, y=w653) -> (x+y=w652:dbl)
            n107 = dll-call lib="C:/Users/Liu Chongyang/Desktop/Hopping_WangYunong/NextXYPos.dll" fn="?ModifyNextPos@@YAHNNNHPAN0PAH11HH00NNN@Z"("xMaxMov"=w652, "yMaxMov"=w649, "xInitPt"=w653, "xPreviousNum"=w648, "calXPos"=w640, "calYPos"=w638, "xCounting"=w636, "yCounting"=w634, "xVel"=w632, "lastZPos"=w630, "preZPos"=w647, "xStepLen"=w628, "yStepLen"=w626, "xInitStepLen"=w646, "yInitStepLen"=w645, "zRisingLimitLen"=w644) -> ("return type"=w641:i32, "calXPos"=w639:dbl, "calYPos"=w637:dbl, "xCounting"=w635:i32, "yCounting"=w633:i32, "xVel"=w631:i32, "preZPos"=w629:i32, "xStepLen"=w627:dbl, "yStepLen"=w625:dbl)  [unwired: 11 in, 2 out]
            n108 = Bundle(w622, w621) -> (→"XY Graph":cluster{dbl[], dbl[]})  [unwired: 1 in]
          }
        }
        n109 = Equal?(x=w111, y=1) -> (x = y?=w113:bool)
        n110 = Or(x=w113, y=w114) -> (x .or. y?=w115:bool)
      }
    }
    frame #5 {
      n111 = VISA Write(VISA resource name=w663, write buffer="MOV A 0\nMOV B 0\nMOV C 0\n", error in (no error)=w662) -> (VISA resource name out=w660:refnum<visa-resource-name>, error out=w659:errorcluster)  [unwired: 1 out]
      n112 = Wait (ms)(milliseconds to wait=u32 100) -> ()  [unwired: 1 out]
    }
    frame #6 {
      n113 = VISA Write(VISA resource name=w672, write buffer="ERR?\n", error in (no error)=w671) -> (VISA resource name out=w669:refnum<visa-resource-name>, error out=w668:errorcluster)  [unwired: 1 out]
      n114 = VISA Read(VISA resource name=w669, byte count=u32 128, error in (no error)=w668) -> (VISA resource name out=w667:refnum<visa-resource-name>, read buffer=w664:string, error out=w666:errorcluster)  [unwired: 1 out]
      n115 = local write "RoughXYZErr?"(w664) -> ()
      n116 = VISA Close(VISA resource name=w667, error in (no error)=w666) -> ()  [unwired: 1 out]
    }
  }
